vi "show_measure (SubVI).vi"(10 "Data in":T1) -> (0 "Z element out":dbl, 1 "Y element out":dbl, 2 "X element out":dbl)   [LabVIEW 2015]
uses:
  data_typedef.ctl
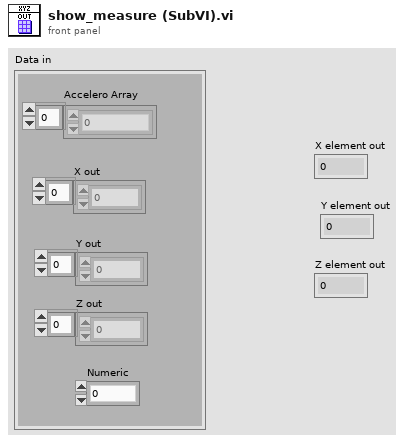
[diagram p1: front panel]
types:
  T1 = typedef "data_typedef.ctl" = cluster{"Accelero Array":dbl[], "Z out":dbl[], "Y out":dbl[], "X out":dbl[], "Numeric":i32}
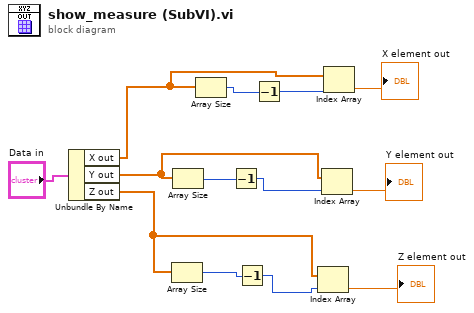
[diagram p0: block diagram]
diagram:
  n1 = Unbundle By Name("Data in") -> ("X out"=w4:dbl[], "Y out"=w3:dbl[], "Z out"=w2:dbl[])
  n2 = Array Size(array=w2) -> (size(s)=w12:i32)
  n3 = Array Size(array=w3) -> (size(s)=w13:i32)
  n4 = Array Size(array=w4) -> (size(s)=w11:i32)
  n5 = Decrement(x=w13) -> (x-1=w9:i32)
  n6 = Decrement(x=w12) -> (x-1=w8:i32)
  n7 = Decrement(x=w11) -> (x-1=w10:i32)
  n8 = Index Array(array=w2, index=w8) -> (element=→"Z element out":dbl)
  n9 = Index Array(array=w3, index=w9) -> (element=→"Y element out":dbl)
  n10 = Index Array(array=w4, index=w10) -> (element=→"X element out":dbl)
